vi "Determine Failure Action UT Main.vi"(5 "Generate Failure Action Change":bool, 6 "Requested Action":T3, 7 "Create Queue":bool, 10 "Failure Action Change Event References in":T1, 11 "Assert Message in":T2) -> (2 "Failure Action Change Event References out":T1, 3 "Assert Message out":T2)   [LabVIEW 2016]
uses:
  Core/Assert API Components/Log Assert Core Components/Event Transmission/Failure Action Change Event Reference.ctl
  Core/Assert API Components/Failure Actions.ctl
  Core/Assert API Components/Message Data.ctl
  Core/Assert API Components/VI References.ctl
  Core/Assert API Components/Log Assert Core Components/Log Assert Core.lvlib
  Core/Assert API Components/Assert API Components.lvlib
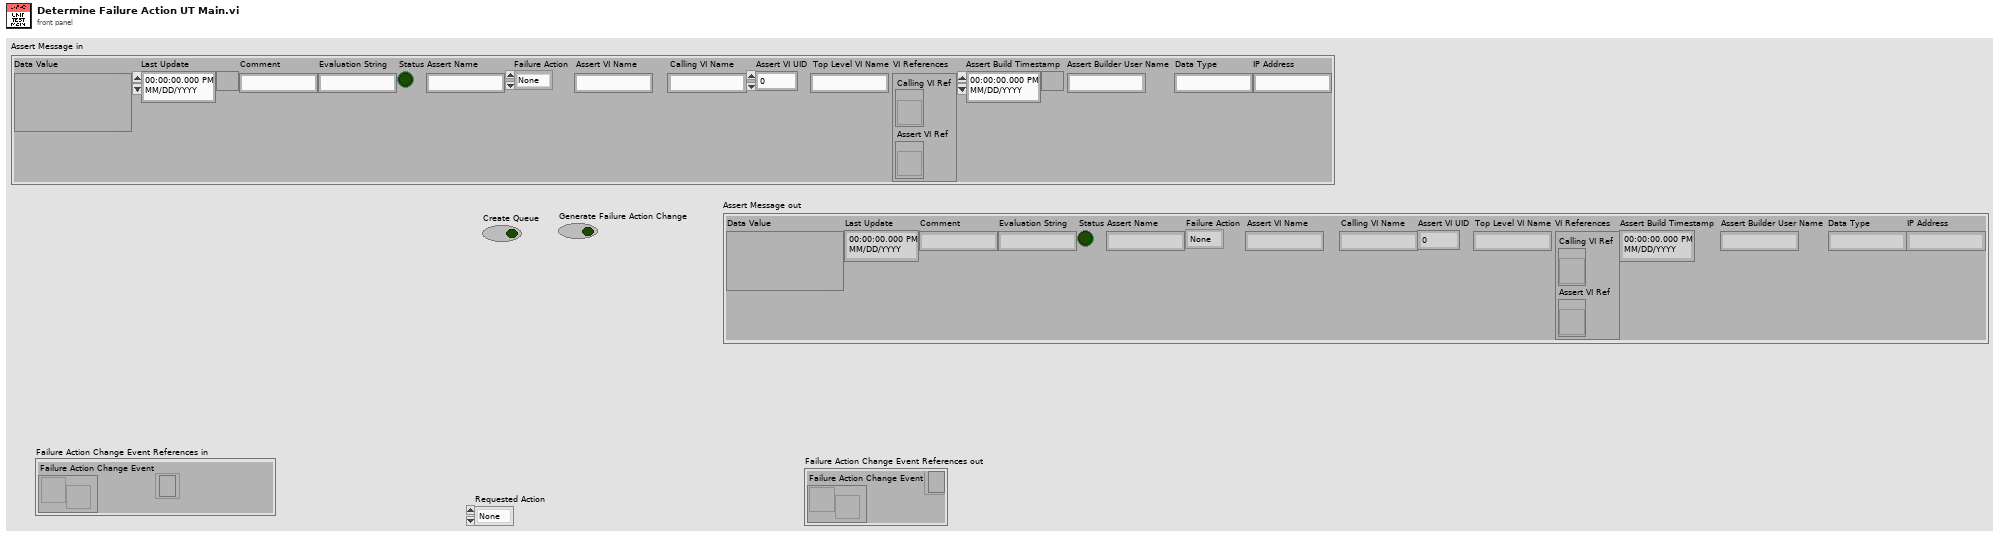
[diagram p1: front panel]
types:
  T1 = typedef "Assert API Components.lvlib/Log Assert Core.lvlib/Failure Action Change Event Reference.ctl" = cluster{"Failure Action Change Event":refnum<user-event>, "Event Registration Refnum":refnum<event-registration>}
  T2 = typedef "Assert API Components.lvlib/Message Data.ctl" = cluster{"Data Value":variant, "Last Update":timestamp, "Comment":string, "Evaluation String":string, "Status":bool, "Assert Name":string, "Failure Action":T3, "Assert VI Name":string, "Calling VI Name":string, "Assert VI UID":i32, "Top Level VI Name":string, "VI References":T4, "Assert Build Timestamp":timestamp, "Assert Builder User Name":string, "Data Type":string, "IP Address":string}
  T3 = typedef "Assert API Components.lvlib/Failure Actions.ctl" = enum16{"None", "Log To File", "Pause Execution", "Abort Execution"}
  T4 = typedef "Assert API Components.lvlib/VI References.ctl" = cluster{"Calling VI Ref":refnum<vi>, "Assert VI Ref":refnum<vi>}
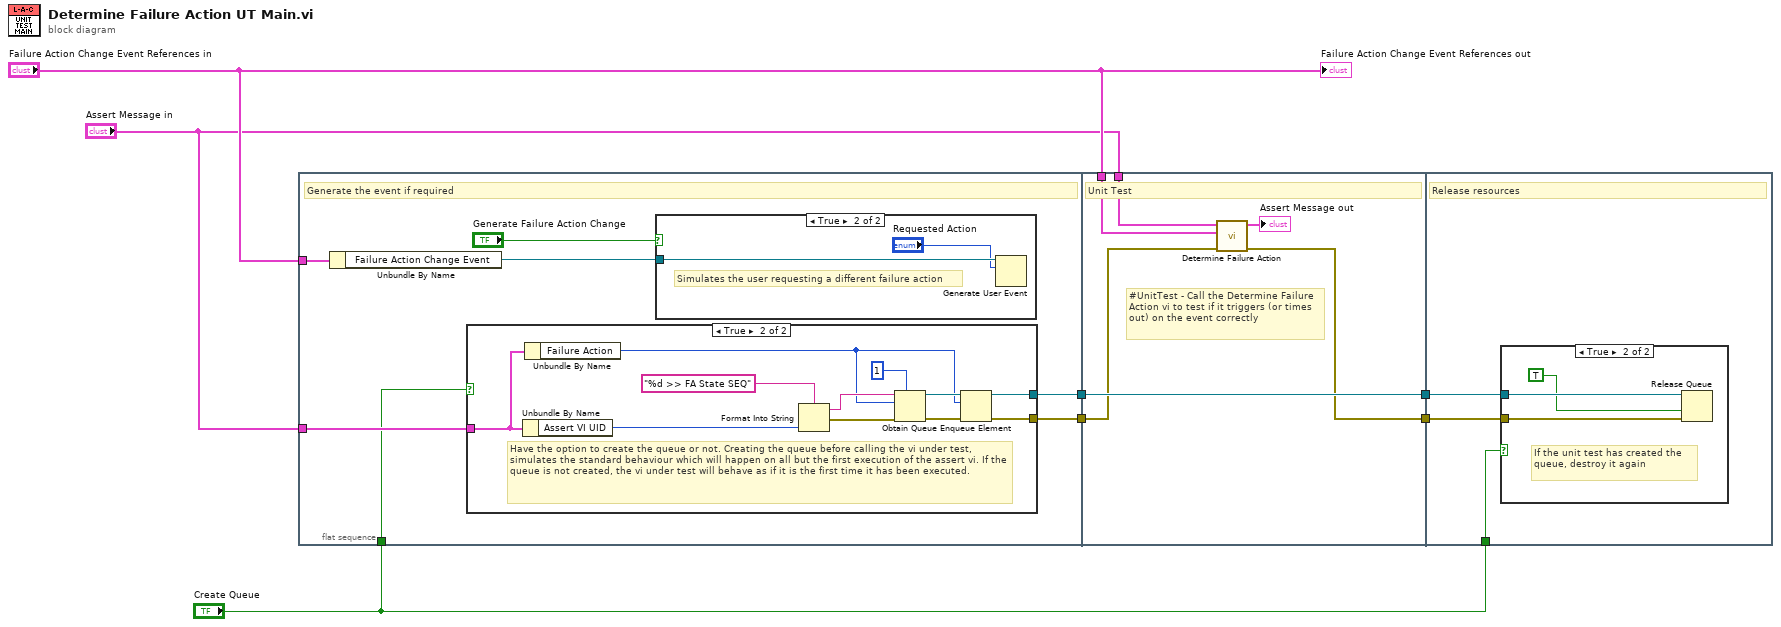
[diagram p0: block diagram]
diagram:
  n1 = flat-sequence {
    tunnel: "Failure Action Change Event References in" -> [w14]
    tunnel: "Assert Message in" -> [w11]
    tunnel: [w10] -> w5
    tunnel: [w9] -> w4
    tunnel: "Create Queue" -> [w8]
    tunnel: "Failure Action Change Event References in" -> [w33]
    tunnel: "Assert Message in" -> [w31]
    tunnel: w5 -> [w30]
    tunnel: w4 -> [w29]
    tunnel: [w30] -> w3
    tunnel: [w28] -> w2
    tunnel: w3 -> [w36]
    tunnel: w2 -> [w35]
    tunnel: "Create Queue" -> [w34]
    frame #0 {
      # "Generate the event if required"
      n2 = Unbundle By Name(w14) -> ("Failure Action Change Event"=w13:refnum<user-event>)
      n3 = case shown="True" w8 {
        tunnel: w11 -> [_ w18]
        tunnel: [_ w16] -> w10
        tunnel: [_ w15] -> w9
        frame False {
        }
        frame True {
          # "Have the option to create the queue or not. Creating the queue before calling the vi under test, simulates the standard behaviour which will happen on all but the first execution of the assert vi. If the queue is not created, the vi under test will behave as if it is the first time it has been executed."
          n4 = Unbundle By Name(w18) -> ("Assert VI UID"=w21:i32)
          n5 = Unbundle By Name(w18) -> ("Failure Action"=w17:T3)
          n6 = Format Into String(format string="%d >> FA State SEQ" ("string"), w21) -> (resulting string=w23:string, error out=w22:errorcluster)  [unwired: 2 in]
          n7 = Obtain Queue(max queue size (-1, unlimited)=1, name (unnamed)=w23, element data type=w17, error in (no error)=w22) -> (queue out=w20:refnum<queue>, error out=w19:errorcluster)  [unwired: 1 in, 1 out]
          n8 = Enqueue Element(queue=w20, element=w17, error in (no error)=w19) -> (queue out=w16:refnum<queue>, error out=w15:errorcluster)  [unwired: 1 in, 1 out]
        }
      }
      n9 = case shown="True" "Generate Failure Action Change" {
        tunnel: w13 -> [_ w27]
        frame False {
        }
        frame True {
          # "Simulates the user requesting a different failure action"
          n10 = Generate User Event(user event=w27, event data cluster="Requested Action") -> ()  [unwired: 2 in, 2 out]
        }
      }
    }
    frame #1 {
      # "#UnitTest - Call the Determine Failure Action vi to test if it triggers (or times out) on the event correctly"
      # "Unit Test"
      n11 = call "Determine Failure Action.vi"("error in (no error)"=w29, "Failure Action Change Event References"=w33, "Assert Message in"=w31) -> ("error out"=w28:errorcluster, "Assert Message out"=→"Assert Message out":T2)  [unwired: 7 in]
    }
    frame #2 {
      # "Release resources"
      n12 = case shown="True" w34 {
        tunnel: w36 -> [_ w39]
        tunnel: w35 -> [_ w38]
        frame False {
        }
        frame True {
          # "If the unit test has created the queue, destroy it again"
          n13 = Release Queue(queue=w39, force destroy? (F)=TRUE, error in (no error)=w38) -> ()  [unwired: 3 out]
        }
      }
    }
  }
  "Failure Action Change Event References out" <- "Failure Action Change Event References in"
